vi "Match_Flow_meters.vi"() -> ()   [LabVIEW 2016]
uses:
  <userlib>/Fluigent/Fluigent MFCS/FluigentMFCS_Full.llb/MFCS_EZ Detect.vi
  <userlib>/Fluigent/Fluigent MFCS/FluigentMFCS_Full.llb/MFCS_EZ Initialization.vi
  Globals/PressuresGlobal.vi
panel:
  out "Current Flow Rates":dbl[](array[numeric])
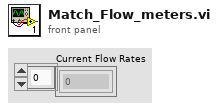
[diagram p1: front panel]
types:
  T1 = typedef "_EZmfcsSN.ctl" = u16
  T2 = typedef "_EZmfcsRefNum.ctl" = refnum<k1>
  T3 = enum16{"Release", "Create", "Send", "Wait", "Cancel"}
  T4 = cluster{"Flowboards":enum16{"A", "B", "C"}[], "Channels":enum16{"1", "2", "3", "4", "5", "6", "7", "8"}[], "States":bool[]}
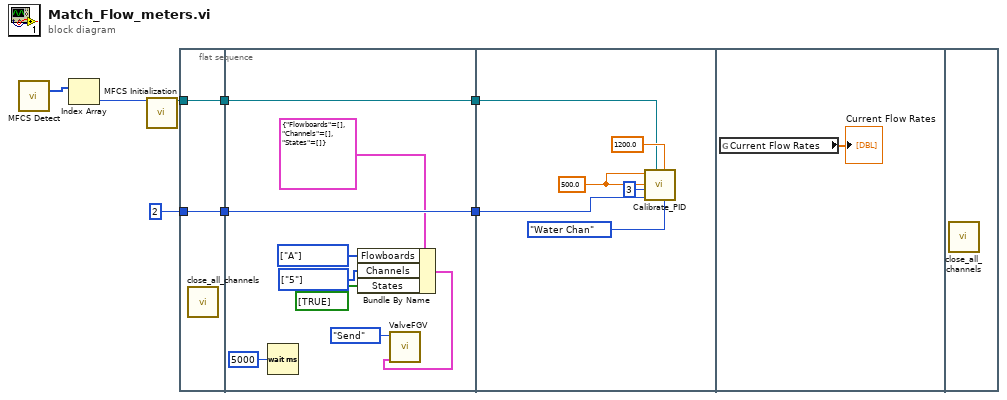
[diagram p0: block diagram]
diagram:
  n1 = call-poly <userlib>:"MFCS Detect.vi"() -> ("[SN MFCS_EZ]"=w8:T1[])  [unwired: 14 in, 1 out]
  n2 = Index Array(array=w8) -> (element=w7:T1)  [unwired: 1 in]
  n3 = call-poly <userlib>:"MFCS Initialization.vi"("SN MFCS_EZ"=w7) -> ("MFCS_EZ"=w6:T2)  [unwired: 12 in, 2 out]
  n4 = flat-sequence {
    tunnel: i16 2 ("Odor Mix Pressure Channel") -> [w9]
    tunnel: w6 -> [w10]
    tunnel: [w10] -> w2
    tunnel: [w9] -> w1
    tunnel: [w19] -> w4
    tunnel: [w18] -> w3
    tunnel: w2 -> [w19]
    tunnel: w1 -> [w18]
    tunnel: w4 -> [w23]
    tunnel: w3 -> [w21]
    frame #0 {
      n5 = call "close_all_channels.vi"() -> ()  [unwired: 12 in]
    }
    frame #1 {
      w15 = enum16{"1", "2", "3", "4", "5", "6", "7", "8"}[] [enum."5"] items=["1", "2", "3", "4", "5", "6", "7", "8"] ("Channels")
      w14 = enum16{"A", "B", "C"}[] [enum."A"] items=["A", "B", "C"] ("Flowboards")
      n6 = Wait (ms)(milliseconds to wait=u32 5000) -> ()  [unwired: 1 out]
      n7 = Bundle By Name(cluster=T4 {"Flowboards"=[], "Channels"=[], "States"=[]} ("Valve Data"), "Flowboards"=w14, "Channels"=w15, "States"=bool[] [TRUE]) -> (w12:T4)
      n8 = call "ValveFGV.vi"("Valve Data"=w12, "Action"=T3."Send") -> ()  [unwired: 6 in, 4 out]
    }
    frame #2 {
      w22 = 500.0 ("Ftot Setpoint")
      n9 = call "Calibrate_PID.vi"("Which Channel To Control"=enum16{"Odor Chan", "Water Chan", "Both"}."Water Chan", "F1 Stability Threshold"=1200.0, "MFCS_EZ"=w23, "Water Mix Pressure Channel"=w21, "Odor Mix Pressure Channel"=i16 3, "Ftot Setpoint"=w22, "F1 Setpoint"=w22) -> ()  [unwired: 3 in, 2 out]
    }
    frame #3 {
      n10 = global read "PressuresGlobal.vi" "Current Flow Rates"() -> (→"Current Flow Rates":dbl[])
    }
    frame #4 {
      n11 = call "close_all_channels.vi"() -> ()  [unwired: 12 in]
    }
  }
